vi "XIPIN_AXI4-Stream_Accelerator_Adapter_2_1.vi"   [LabVIEW 2017]
doc: "The Xilinx Accelerator Adapter LogiCCORE provides flexible interface for AXI4-Stream interface to Xilinx BRAM/FIFO interface towards accelerators.\n------------------------------------\n<b>Need License</b> : No\n<b>Interface</b> : AXI4 AXI4-Stream"
uses:
  <vilib>/rvi/XilinxIP/XIPIN_XNode/niFpgaXIPIN.xnode
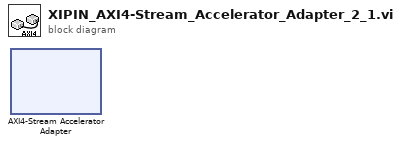
[diagram p0: block diagram]
diagram:
  n1 = xnode ("AXI4-Stream Accelerator Adapter")() -> ()
